vi "Gear State Machine.vi"(8 "Lower Limit Switch Name":string, 9 "Upper Limit Switch Name":string, 10 "Lower Limit Button":bool, 11 "Upper Limit Button":bool) -> ()   [LabVIEW 2016]
uses:
  <vilib>/Rock Robotics/Network Tables/NT Write Boolean.vi
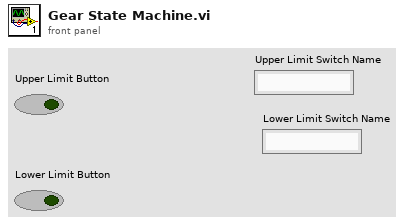
[diagram p1: front panel]
types:
  T1 = typedef "WPI_SwitchDevRef.ctl" = cluster{"DevStatus":errorcluster, "DIO Channel":T2, "CntIndex":T3, "Normally Closed":bool}
  T2 = typedef "FPGA_DIOChannel.ctl" = enum8{"DIO 0", "DIO 1", "DIO 2", "DIO 3", "DIO 4", "DIO 5", "DIO 6", "DIO 7", "DIO 8", "DIO 9", "DIO MXP 0", "DIO MXP 1", "DIO MXP 2", "DIO MXP 3", "DIO MXP 4", "DIO MXP 5", "DIO MXP 6", "DIO MXP 7", "DIO MXP 8", "DIO MXP 9", "DIO MXP 10", "DIO MXP 11", "DIO MXP 12", "DIO MXP 13", "DIO MXP 14", "DIO MXP 15", "SPI Port CS1", "SPI Port CS2", "SPI Port CS3", "SPI Port MISO", "SPI Port MOSI", "Invalid"}
  T3 = typedef "FPGA_CounterCtrSystemIndex.ctl" = enum8{"Ctr 0", "Ctr 1", "Ctr 2", "Ctr 3", "Ctr 4", "Ctr 5", "Ctr 6", "Ctr 7", "Invalid"}
  T4 = enum16{"Start", "Go To Upper", "Go To Lower", "Finish"}
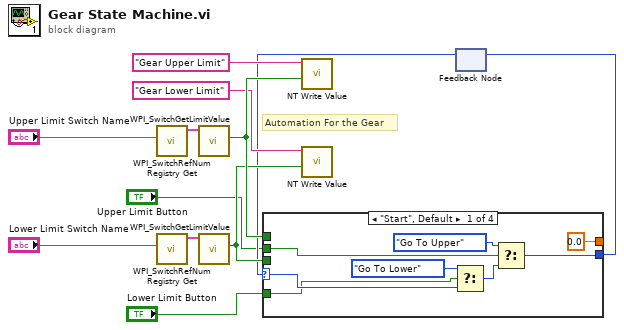
[diagram p0: block diagram]
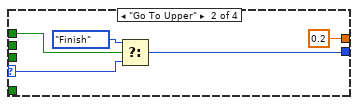
[diagram p2: hidden frame]
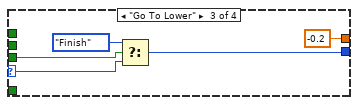
[diagram p3: hidden frame]
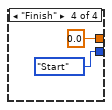
[diagram p4: hidden frame]
diagram:
  # "Automation For the Gear"
  n1 = call <vilib>:"WPI_SwitchRefNum Registry Get.vi"("refnum name"="Upper Limit Switch Name") -> ("SwitchDevRef"=w5:T1)  [unwired: 9 in, 1 out]
  n2 = call <vilib>:"WPI_SwitchRefNum Registry Get.vi"("refnum name"="Lower Limit Switch Name") -> ("SwitchDevRef"=w6:T1)  [unwired: 9 in, 1 out]
  n3 = call <vilib>:"WPI_SwitchGetLimitValue.vi"("SwitchDevRef"=w5) -> ("Switch Pressed"=w12:bool)  [unwired: 8 in, 2 out]
  n4 = call <vilib>:"WPI_SwitchGetLimitValue.vi"("SwitchDevRef"=w6) -> ("Switch Pressed"=w9:bool)  [unwired: 8 in, 2 out]
  n5 = call-poly <vilib>:"NT Write Value.vi"("Boolean"=w12, "Name"="Gear Upper Limit") -> ()  [unwired: 9 in, 1 out]
  n6 = call-poly <vilib>:"NT Write Value.vi"("Boolean"=w9, "Name"="Gear Lower Limit") -> ()  [unwired: 9 in, 1 out]
  n7 = feedback #1() -> (w8:T4)  [unwired: 1 in]
  n8 = case shown="\"Start\", Default" w8 {
    selector: w8 -> [w16 w25 w29 _]
    tunnel: [w19 w24 w30 T4."Start" ("t")] -> w7
    tunnel: w12 -> [_ w23 _ _]
    tunnel: w9 -> [_ _ w28 _]
    tunnel: [0.0 0.2 -0.2 0.0] -> _
    tunnel: "Upper Limit Button" -> [w14 _ _ _]
    tunnel: "Lower Limit Button" -> [w13 _ _ _]
    frame "Start", Default {
      n9 = Select(t=T4."Go To Lower", s=w13, f=w16) -> (s? t:f=w18:T4)
      n10 = Select(t=T4."Go To Upper", s=w14, f=w18) -> (s? t:f=w19:T4)
    }
    frame "Go To Upper" {
      n11 = Select(t=T4."Finish", s=w23, f=w25) -> (s? t:f=w24:T4)
    }
    frame "Go To Lower" {
      n12 = Select(t=T4."Finish", s=w28, f=w29) -> (s? t:f=w30:T4)
    }
    frame "Finish" {
    }
  }
  n13 = feedback-in #1(w7) -> ()
